vi "AlliGator Get LaVision .set File Path.vi"(8 "Error In":errorcluster, 11 "Gate Image Folder Path":path) -> (0 "Error Out":errorcluster, 3 ".set File Path":path)   [LabVIEW 2021, in "AlliGator Files.lvlib"]
doc: "Tries to extract FLI dataset metadata corresponding to one of LaVision formats."
uses:
  AlliGator Files.lvlib
panel:
  # "see the AlliGator License on the block diagram (Ctrl+E or Window:Show Block Diagram)"
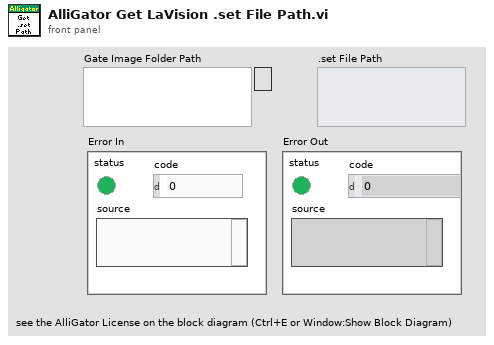
[diagram p1: front panel]
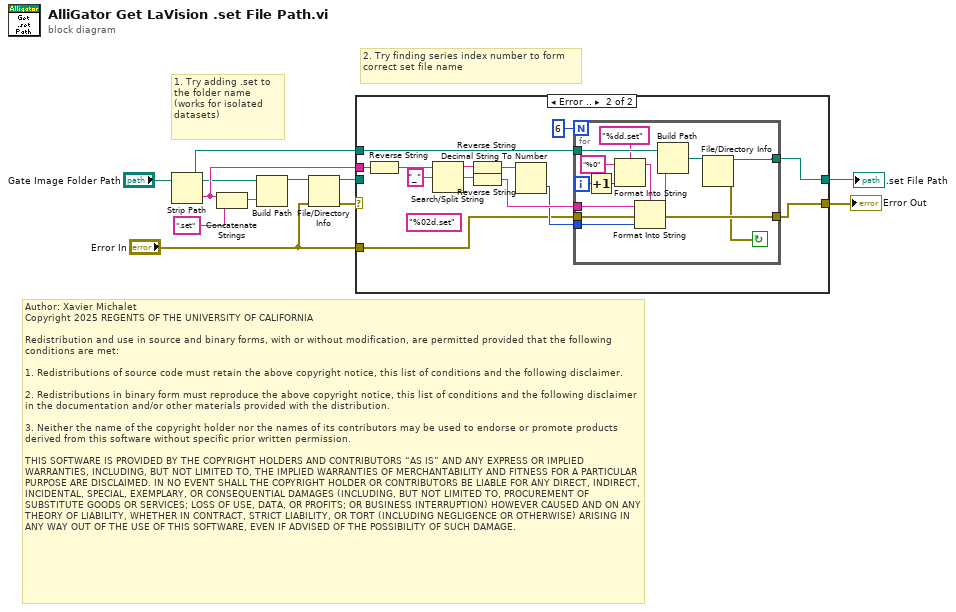
[diagram p0: block diagram]
diagram:
  # "Author: Xavier Michalet\nCopyright 2025 REGENTS OF THE UNIVERSITY OF CALIFORNIA\n\nRedistribution and use in source and binary forms, with or without modification, are permitted provided that the following conditions are met:\n\n1. Redistributions of source code must retain the above copyright notice, this list of conditions and the following disclaimer.\n\n2. Redistributions in binary form must reproduce the above copyright notice, this list of conditions and the following disclaimer in the documentation and/or other materials provided with the distribution.\n\n3. Neither the name of the copyright holder nor the names of its contributors may be used to endorse or promote products derived from this software without specific prior written permission.\n\nTHIS SOFTWARE IS PROVIDED BY THE COPYRIGHT HOLDERS AND CONTRIBUTORS “AS IS” AND ANY EXPRESS OR IMPLIED WARRANTIES, INCLUDING, BUT NOT LIMITED TO, THE IMPLIED WARRANTIES OF MERCHANTABILITY AND FITNESS FOR A PARTICULAR PURPOSE ARE DISCLAIMED. IN NO EVENT SHALL THE COPYRIGHT HOLDER OR CONTRIBUTORS BE LIABLE FOR ANY DIRECT, INDIRECT, INCIDENTAL, SPECIAL, EXEMPLARY, OR CONSEQUENTIAL DAMAGES (INCLUDING, BUT NOT LIMITED TO, PROCUREMENT OF SUBSTITUTE GOODS OR SERVICES; LOSS OF USE, DATA, OR PROFITS; OR BUSINESS INTERRUPTION) HOWEVER CAUSED AND ON ANY THEORY OF LIABILITY, WHETHER IN CONTRACT, STRICT LIABILITY, OR TORT (INCLUDING NEGLIGENCE OR OTHERWISE) ARISING IN ANY WAY OUT OF THE USE OF THIS SOFTWARE, EVEN IF ADVISED OF THE POSSIBILITY OF SUCH DAMAGE."
  # "2. Try finding series index number to form correct set file name"
  # "1. Try adding .set to the folder name (works for isolated datasets)"
  n1 = Strip Path(path="Gate Image Folder Path") -> (stripped path=w1:path, name=w2:string)
  n2 = Concatenate Strings(w2, ".set" ("string")) -> (w9:string)
  n3 = Build Path(base path=w1, name or relative path=w9) -> (appended path=w8:path)
  n4 = File/Directory Info(path=w8, error in="Error In") -> (path out=w6:path, error out=w7:errorcluster)  [unwired: 5 out]
  n5 = case shown="Error .." w7 {
    selector: w7 -> [w12 _]
    tunnel: w6 -> [w13 _]
    tunnel: [w13 w15] -> w5
    tunnel: [w12 w16] -> w4
    tunnel: "Error In" -> [_ w18]
    tunnel: w2 -> [_ w26]
    tunnel: w1 -> [_ w17]
    frame No Error {
    }
    frame Error {
      (unwired) "%02d.set" ("format string")
      n6 = Reverse String(1:w26) -> (0:w24:string)
      n7 = Search/Split String(string=w24, search string/char (-)="_") -> (substring before match=w23:string, match + rest of string=w21:string)  [unwired: 1 in, 1 out]
      n8 = Reverse String(1:w23) -> (0:w22:string)
      n9 = Reverse String(1:w21) -> (0:w20:string)
      n10 = Decimal String To Number(string=w22) -> (number=w19:i32)  [unwired: 2 in, 1 out]
      n11 = for {
        N: 6 -> [_]
        tunnel: w20 -> [w40]
        tunnel: w19 -> [w39]
        tunnel: w18 -> [w38]
        tunnel: [w35] -> w16
        tunnel: w17 -> [w37]
        tunnel: [w33] -> w15
        i -> [w31]
        stop <- w32 continue-if-true
        n12 = Increment(x=w31) -> (x+1=w30:i32)
        n13 = Format Into String(format string="%dd.set", initial string="%0", w30) -> (resulting string=w27:string)  [unwired: 1 in, 1 out]
        n14 = Format Into String(format string=w27, initial string=w40, error in=w38, w39) -> (resulting string=w36:string, error out=w35:errorcluster)
        n15 = Build Path(base path=w37, name or relative path=w36) -> (appended path=w34:path)
        n16 = File/Directory Info(path=w34) -> (path out=w33:path, error out=w32:errorcluster)  [unwired: 1 in, 5 out]
      }
    }
  }
  ".set File Path" <- w5
  "Error Out" <- w4
